vi "DAQFileIO.vi"(6 "Aquire Data":bool, 8 "error in (no error)":errorcluster, 9 "File Path In":path, 10 "Names":string[](array[string])=["Resistance (Ohms)", "Ethanol (%)", "RH (%)", "Temp (C)", "MFC A", "MFC B"], 11 "data":waveform(dbl)[](array[waveform])) -> (0 "error out":errorcluster, 1 "file path out":path)   [LabVIEW 2019, in "DAQ.lvclass"]
uses:
  DAQ.lvclass
  <vilib>/Waveform/WDTOps.llb/WDT Append Waveforms DBL.vi
panel:
  in  "Names":string[](array[string])=["Resistance (Ohms)", "Ethanol (%)", "RH (%)", "Temp (C)", "MFC A", "MFC B"]
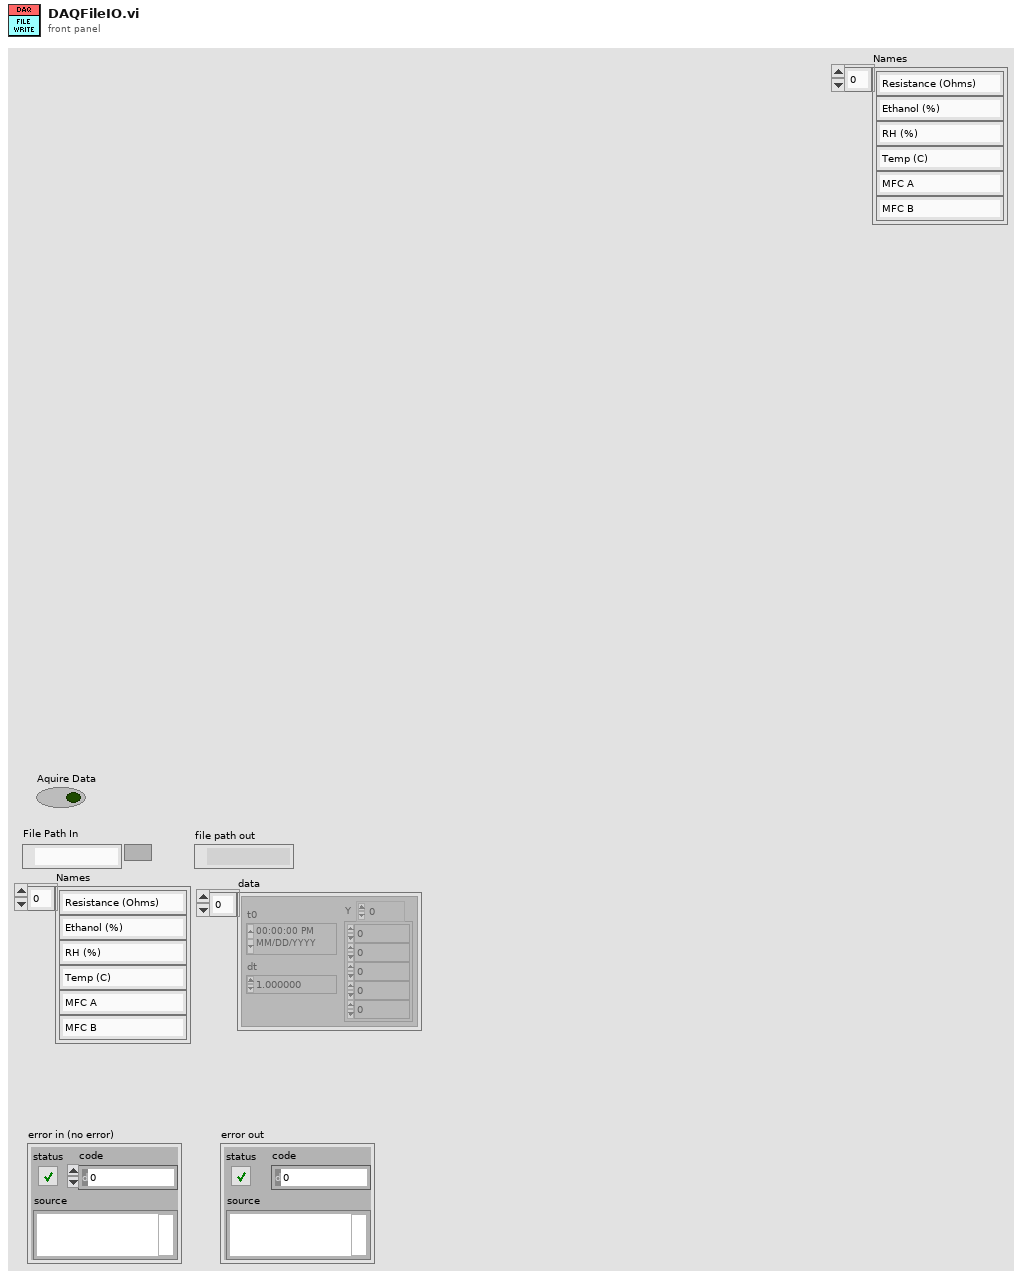
[diagram p1: front panel]
types:
  T1 = enum16{"open", "open or create", "create or replace", "create", "open (read-only)"}
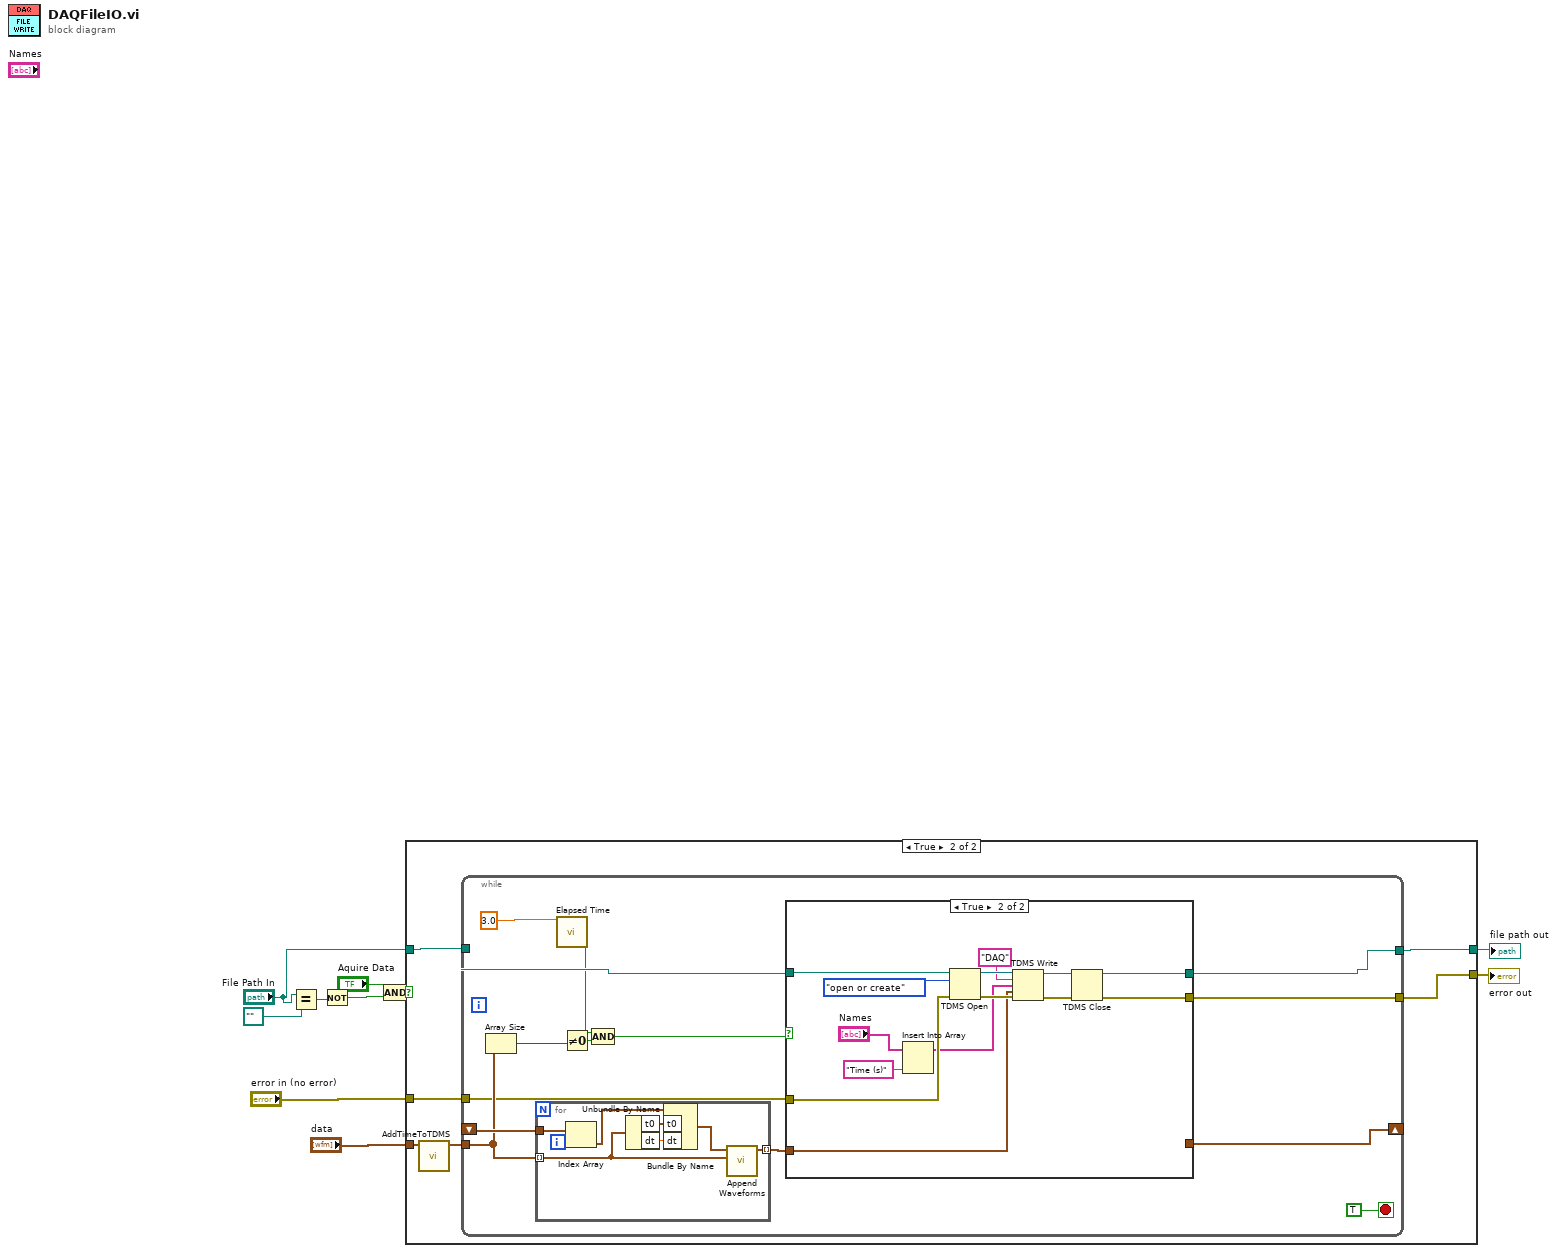
[diagram p0: block diagram]
diagram:
  n1 = Equal?(x="File Path In", y=path "") -> (x = y?=w3:bool)
  n2 = Not(x=w3) -> (.not. x?=w9:bool)
  n3 = Compound Arithmetic op=AND("Aquire Data", w9) -> (w2:bool)
  n4 = case shown="True" w2 {
    tunnel: [w12 w17] -> w8
    tunnel: "File Path In" -> [w12 w18]
    tunnel: [w11 w16] -> w7
    tunnel: "error in (no error)" -> [w11 w15]
    tunnel: "data" -> [_ w14]
    frame False {
    }
    frame True {
      n5 = call "AddTimeToTDMS.vi"("data"=w14) -> ("Data out"=w13:waveform(dbl)[])  [unwired: 9 in, 1 out]
      n6 = while {
        tunnel: w13 -> [w20]
        tunnel: w18 -> [w32]
        tunnel: [w31] -> w17
        tunnel: w15 -> [w19]
        tunnel: [w30] -> w16
        shift-right: [w23] -> _
        shift-left: _ -> [w22]
        stop <- TRUE stop-if-true
        n7 = Array Size(array=w20) -> (size(s)=w28:i32)
        n8 = for {
          tunnel: w22 -> [w38]
          tunnel: [w40] -> w21 mode=indexing
          tunnel: w20 -> [w33] mode=indexing
          i -> [w39]
          n9 = Index Array(array=w38, index=w39) -> (element=w36:waveform(dbl))
          n10 = Unbundle By Name(w33) -> ("t0"=w37:timestamp, "dt"=w34:dbl)
          n11 = Bundle By Name(cluster=w36, "t0"=w37, "dt"=w34) -> (w35:waveform(dbl))
          n12 = call-poly <vilib>:"Append Waveforms.vi"("waveform B"=w33, "waveform A"=w35) -> ("waveform out"=w40:waveform(dbl))  [unwired: 8 in, 1 out]
        }
        n13 = call "Elapsed Time"("Time Target (s)"=3.0) -> ("Time has Elapsed"=w26:bool)  [unwired: 11 in, 7 out]
        n14 = Not Equal To 0?(x=w28) -> (x != 0?=w27:bool)
        n15 = Compound Arithmetic op=AND(w26, w27) -> (w25:bool)
        n16 = case shown="True" w25 {
          tunnel: w32 -> [w43 w57]
          tunnel: [w43 w52] -> w31
          tunnel: [w41 w51] -> w30
          tunnel: w19 -> [w41 w50]
          tunnel: w21 -> [w42 w47]
          tunnel: [w42 _] -> w23
          frame False {
          }
          frame True {
            n17 = Insert Into Array(array="Names", new element="Time (s)" ("new element/subarray")) -> (w44:string[])  [unwired: 1 in]
            n18 = TDMS Open(8:w50, 10:T1."open or create" ("operation (0:open)"), 11:w57) -> (0:w55:errorcluster, 3:w56:refnum<k34>)  [unwired: 4 in]
            n19 = TDMS Write(0:w56, 5:"DAQ" ("group name in (Untitled)"), 7:w44, 9:w47, 11:w55) -> (4:w53:refnum<k34>, 15:w54:errorcluster)  [unwired: 1 in, 2 out]
            n20 = TDMS Close(8:w54, 11:w53) -> (0:w51:errorcluster, 3:w52:path)
          }
        }
      }
    }
  }
  "file path out" <- w8
  "error out" <- w7
